vi "weight test s.vi"() -> ()   [LabVIEW 2019]
uses:
  Timer Delay/Timers.lvlib
panel:
  out "Q":T1 {"Q1g" format="%#.1f"; "Q60" format="%#.1f"; "1 час" format="%#.0f"; "Q10" format="%#.1f"; "10 мин" format="%#.0f"; "Q5" format="%#.1f"; "5 мин" format="%#.0f"; "Q10g" format="%#.1f"; "dT 1" format="%#.0f"}
  in  "Reset":bool
  in  "Weight ohaus":dbl caption="Весы"
  out "W1":refnum<vi>
  out "Waveform Chart":cluster{"[0]":dbl}(graph)
  out "Waveform Chart 2":cluster{"[0]":dbl, "[1]":dbl, "[2]":dbl}(graph)
  out "Вес":dbl caption="g"
  # "время 10 g"
  # "(вес за период)"
  # "(расход)"
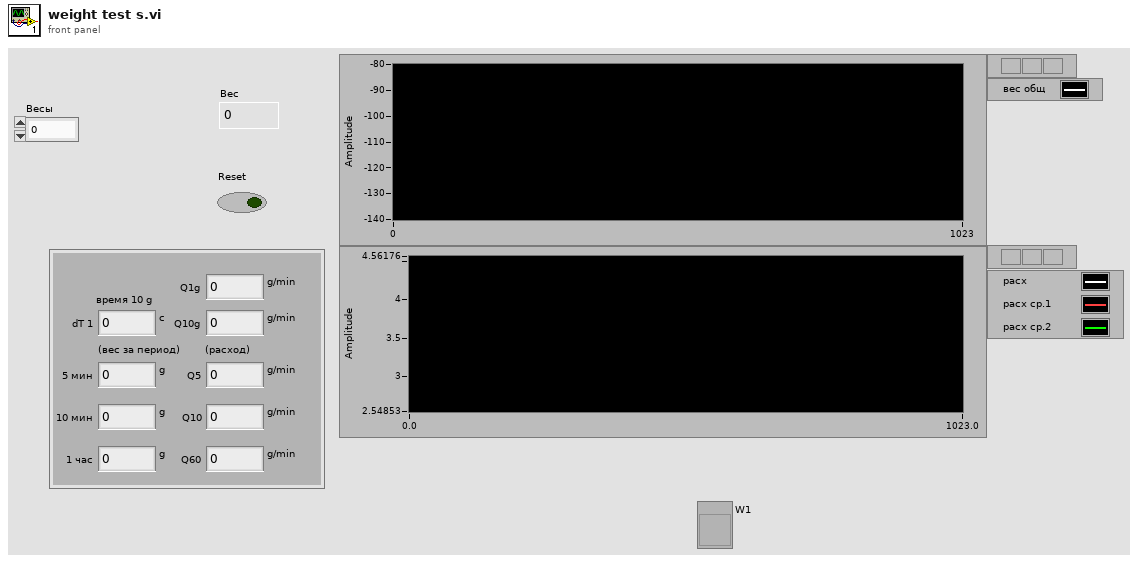
[diagram p1: front panel]
types:
  T1 = cluster{"Q1g":dbl, "Q10g":dbl, "dT 1":dbl, "Q5":dbl, "5 мин":dbl, "Q10":dbl, "10 мин":dbl, "Q60":dbl, "1 час":dbl}
  T2 = cluster{"Q m":dbl, "Q 1":dbl, "dT 1":dbl, "Q 2":dbl, "dM 2":dbl, "Q 3":dbl, "dM 3":dbl, "Q 4":dbl, "dM 4":dbl}
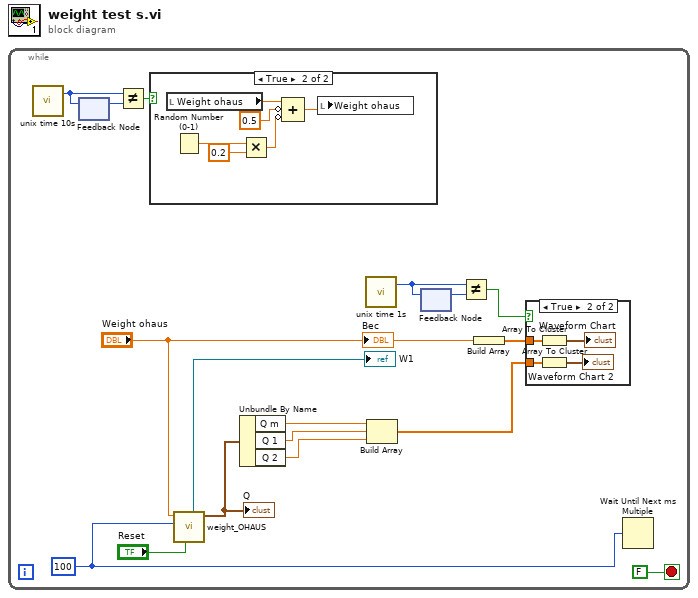
[diagram p0: block diagram]
diagram:
  n1 = while {
    stop <- FALSE stop-if-true
    w5 = u32 100 ("millisecond multiple")
    n2 = call "unix time 10s.vi"() -> ("unix time (ms)"=w8:u64)  [unwired: 2 in, 1 out]
    n3 = feedback #1() -> (w9:u64)  [unwired: 1 in]
    n4 = feedback-in #1(w8) -> ()
    n5 = Not Equal?(x=w8, y=w9) -> (x != y?=w7:bool)
    n6 = case shown="True" w7 {
      frame False {
      }
      frame True {
        n7 = local read "Weight ohaus"() -> (w23:dbl)
        n8 = Random Number (0-1)() -> (number: 0 to 1=w20:dbl)
        n9 = Multiply(x=w20, y=0.2) -> (x*y=w18:dbl)
        n10 = Compound Arithmetic op=ADD(w23, invert 0.5 ("y"), invert w18) -> (w22:dbl)
        n11 = local write "Weight ohaus"(w22) -> ()
      }
    }
    n12 = call "weight_OHAUS.vi"("Reset"="Reset", "Tick"=w5, "PV weight"="Weight ohaus") -> ("Q"=w4:T2, "This VI"=→"W1":refnum<vi>)  [unwired: 7 in]
    "Q" <- w4
    n13 = Unbundle By Name(w4) -> ("Q m"=w3:dbl, "Q 1"=w2:dbl, "Q 2"=w1:dbl)
    n14 = call "unix time 1s.vi"() -> ("unix time (ms)"=w17:u64)  [unwired: 2 in, 1 out]
    n15 = Build Array(w3, w2, w1) -> (w13:dbl[])
    n16 = feedback #2() -> (w16:u64)  [unwired: 1 in]
    n17 = feedback-in #2(w17) -> ()
    n18 = Not Equal?(x=w17, y=w16) -> (x != y?=w15:bool)
    n19 = Build Array("Weight ohaus") -> (w14:dbl[])
    n20 = case shown="True" w15 {
      tunnel: w14 -> [_ w27]
      tunnel: w13 -> [_ w25]
      frame False {
      }
      frame True {
        n21 = Array To Cluster(array=w27) -> (cluster=→"Waveform Chart":cluster{"[0]":dbl})
        n22 = Array To Cluster(array=w25) -> (cluster=→"Waveform Chart 2":cluster{"[0]":dbl, "[1]":dbl, "[2]":dbl})
      }
    }
    n23 = Wait Until Next ms Multiple(millisecond multiple=w5) -> ()  [unwired: 1 out]
    "Вес" <- "Weight ohaus"
  }
